vi "S8300E_CheckSN_auto.vi"() -> ()   [LabVIEW 2011]
panel:
  out "UUT SN":string
  out "UUT SN List":string
  out "CMD-LIST":cluster{string, string, string, string}[](array[cluster])
  out "log msg":string
  out "VISA resource name out":refnum<visa-resource-name>
  out "BEGIN TIME":u32
  out "進行狀況":string
  # "Error Code:SN-BIOS\nError Code:SN-DMI"
  # "S8300E Program SN (接UART COM9)"
  # "2014-12-12"
  # "Step1:Get Serial Number from BIOS Flash\nStep2:Get Serial Number from DMI table"
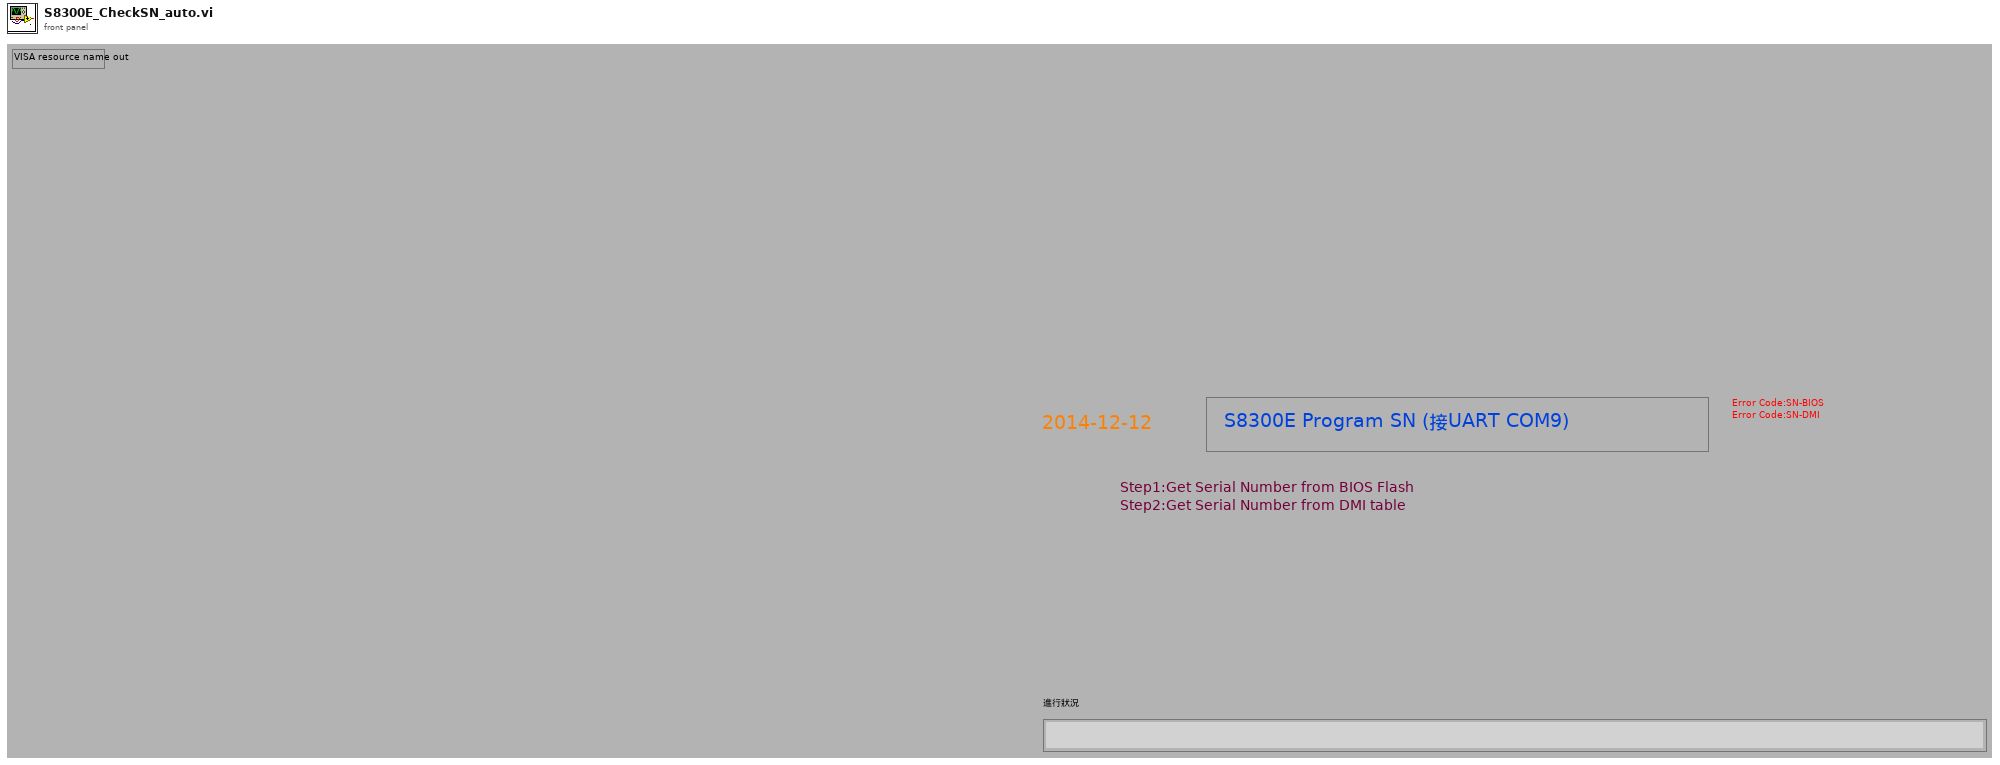
[diagram p1: front panel]
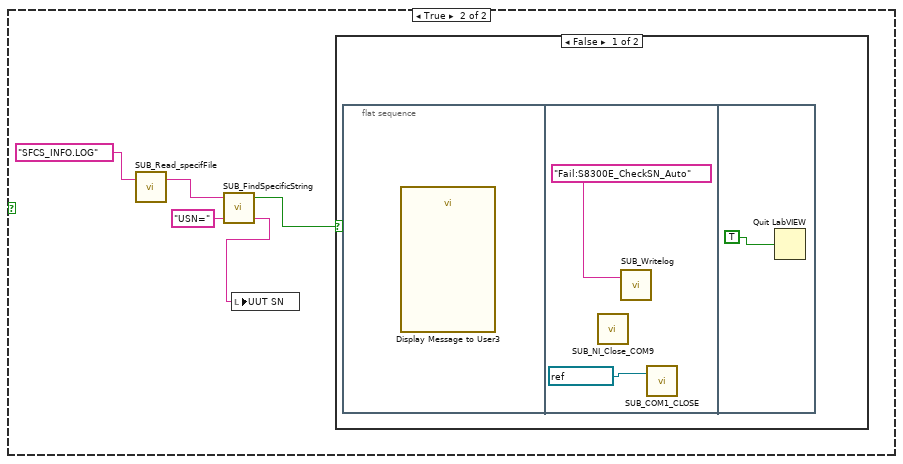
[diagram p3: hidden frame]
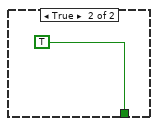
[diagram p8: hidden frame]
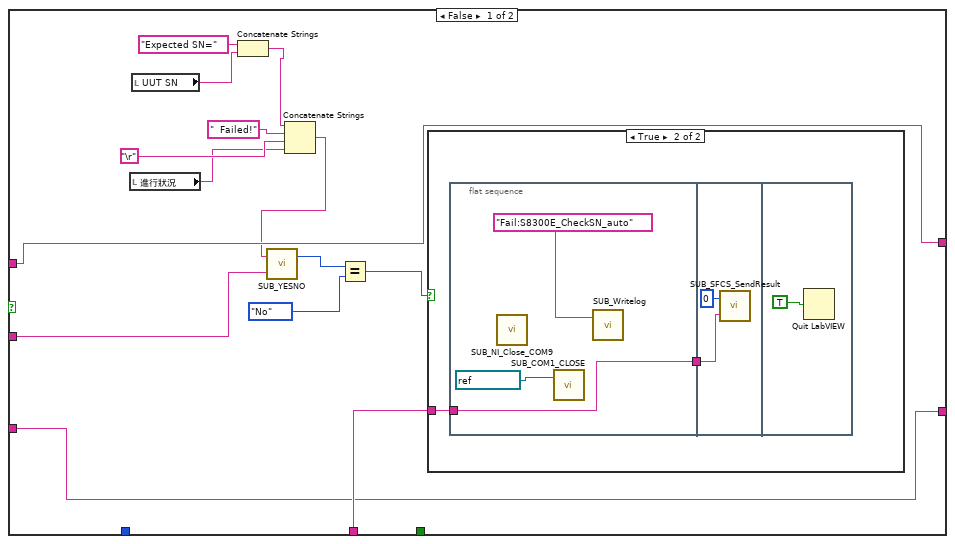
[diagram p9: hidden frame]
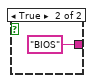
[diagram p11: hidden frame]
diagram:
  n1 = flat-sequence {
    frame #0 {
      n2 = Tick Count (ms)() -> (millisecond timer value=→"BEGIN TIME":u32)
    }
    frame #1 {
      n3 = call "SUB_COM1_CLOSE.vi"("VISA resource name"=refnum<visa-resource-name> "COM9") -> ()  [unwired: 3 in]
      n4 = call "SUB_COM1_CLOSE.vi"("VISA resource name"=refnum<visa-resource-name> "COM9") -> ()  [unwired: 3 in]
      n5 = property on="進行狀況" class="Str"("Blinking"=TRUE) -> ()  [unwired: 2 in, 2 out]
      "進行狀況" <- "進入測試準備中...." ("進行狀況")
      "UUT SN" <- ""
    }
    frame #2 {
      n6 = call "SUB_SearchFile_inFolder.vi"("Search Filename in Folder"="S8300E_sfcs_misc.txt") -> ("File Existing True/Flase"=w7:bool)  [unwired: 1 in]
      n7 = case shown="False" w7 {
        frame False {
          n8 = flat-sequence {
            frame #0 {
              n9 = call "Display Message to User"() -> ()  [unwired: 10 in, 2 out]
            }
            frame #1 {
              n10 = call "SUB_COM1_CLOSE.vi"("VISA resource name"=refnum<visa-resource-name> "COM9") -> ()  [unwired: 3 in]
              n11 = call "SUB_Writelog.vi"("Pass/Fail"="Fail:S8300E_CheckSN_Manual") -> ()  [unwired: 2 in]
            }
            frame #2 {
              n12 = Quit LabVIEW(quit? (T)=TRUE) -> ()
            }
          }
        }
        frame True {
        }
      }
    }
    frame #3 {
      n13 = call "SUB_SearchFile_inFolder.vi"("Search Filename in Folder"="SFCS_INFO.LOG") -> ("File Existing True/Flase"=w12:bool)  [unwired: 1 in]
      n14 = case shown="False" w12 {
        frame False {
          n15 = flat-sequence {
            frame #0 {
              n16 = call "Display Message to User2"() -> ()  [unwired: 10 in, 2 out]
            }
            frame #1 {
              n17 = call "SUB_Writelog.vi"("Pass/Fail"="Fail:S8300E_CheckSN_Auto") -> ()  [unwired: 2 in]
              n18 = call "SUB_NI_Close_COM9.vi"() -> ()  [unwired: 1 in, 1 out]
              n19 = call "SUB_COM1_CLOSE.vi"("VISA resource name"=refnum<visa-resource-name> "COM9") -> ()  [unwired: 3 in]
            }
            frame #2 {
              n20 = Quit LabVIEW(quit? (T)=TRUE ("stop? (T)")) -> ()
            }
          }
        }
        frame True {
          n21 = call "SUB_Read_specifFile.vi"("name or relative path"="SFCS_INFO.LOG") -> ("text"=w20:string)  [unwired: 1 in, 1 out]
          n22 = call "SUB_FindSpecificString.vi"("Find this String"="USN=", "String data"=w20) -> ("before \"; \" string"=w17:string, "Found"=w18:bool)  [unwired: 2 in]
          n23 = local write "UUT SN"(w17) -> ()
          n24 = case shown="False" w18 {
            frame False {
              n25 = flat-sequence {
                frame #0 {
                  n26 = call "Display Message to User3"() -> ()  [unwired: 10 in, 2 out]
                }
                frame #1 {
                  n27 = call "SUB_NI_Close_COM9.vi"() -> ()  [unwired: 1 in, 1 out]
                  n28 = call "SUB_Writelog.vi"("Pass/Fail"="Fail:S8300E_CheckSN_Auto") -> ()  [unwired: 2 in]
                  n29 = call "SUB_COM1_CLOSE.vi"("VISA resource name"=refnum<visa-resource-name> "COM9") -> ()  [unwired: 3 in]
                }
                frame #2 {
                  n30 = Quit LabVIEW(quit? (T)=TRUE ("stop? (T)")) -> ()
                }
              }
            }
            frame True {
            }
          }
        }
      }
    }
    frame #4 {
      n31 = local read "UUT SN"() -> (w26:string)
      n32 = Concatenate Strings("PASSED=", w26) -> (w25:string)
      n33 = Concatenate Strings("PASSED=", w26) -> (w28:string)
      n34 = Concatenate Strings("./ser.sh -w -f  ", w26, "\r") -> (w47:string)
      n35 = Concatenate Strings("./ser.sh -r -f  ", "\r") -> (w43:string)
      n36 = Concatenate Strings("./ser.sh -r -d ", "\r") -> (w40:string)
      n37 = Bundle(w47, "PASSED=", "Set Serial Number to BIOS Flash", "SN-BIOS") -> ()  [unwired: 1 in, 1 out]
      n38 = Bundle(w43, w28, "Get Serial Number from BIOS Flash", "SN-BIOS") -> (w35:cluster{string, string, string, string})  [unwired: 1 in]
      n39 = Bundle(w40, w25, "Get Serial Number from DMI table", "SN-DMI") -> (w34:cluster{string, string, string, string})  [unwired: 1 in]
      n40 = Build Array(w35, w34) -> (→"CMD-LIST":cluster{string, string, string, string}[])
    }
    frame #5 {
      n41 = case shown="True" TRUE {
        frame False {
        }
        frame True {
          n42 = call "SUB_COM9_INIT.vi"("baud rate"=u32 115200) -> ("VISA resource name out"=w53:refnum<visa-resource-name>)  [unwired: 1 in, 1 out]
          "VISA resource name out" <- w53
          n43 = call "SUB_COM1Wrt.vi"("VISA resource name"=w53, "write buffer"="\r") -> ("duplicate VISA resource name"=w50:refnum<visa-resource-name>)  [unwired: 1 in, 1 out]
          n44 = call "SUB_ContinueCom1Read.vi"("Numeric"=1200, "duplicate VISA resource name 2"=w50) -> ()  [unwired: 1 in, 3 out]
        }
      }
    }
    frame #6 {
      n45 = case shown="True" TRUE {
        frame False {
        }
        frame True {
          n46 = while {
            stop <- w65 stop-if-true
            w56 = "\r"
            n47 = Concatenate Strings(w56, w56, w56) -> (w57:string)
            n48 = local read "VISA resource name out"() -> (w58:refnum<visa-resource-name>)
            n49 = call "SUB_COM1Wrt.vi"("VISA resource name"=w58, "write buffer"=w57) -> ("duplicate VISA resource name"=w64:refnum<visa-resource-name>)  [unwired: 1 in, 1 out]
            n50 = Tick Count (ms)() -> (millisecond timer value=w63:u32)
            n51 = call "SUB_READ_COM1_FindString_timeout.vi"("Find this String"="s8300e_func_test#", "Timeout Seccond"=3.0, "Begin time"=w63, "duplicate VISA resource name 2"=w64) -> ("Output String"=w59:string, "Found String"=w60:bool)  [unwired: 1 in, 1 out]
            n52 = case shown="False" w60 {
              tunnel: [w67 TRUE] -> w65
              tunnel: w59 -> [w66 _]
              frame False {
                n53 = call "SUB_YESNO.vi"("Debug View"=w66, "Status"="UART無正確反應!需有S8300E字串") -> ("yes/no"=w70:enum32{"No Selection", "Yes", "No", "None"})  [unwired: 1 in]
                n54 = Equal?(x=w70, y=enum32{"No Selection", "Yes", "No", "None"}."No") -> (x = y?=w68:bool)
                n55 = case shown="True" w68 {
                  tunnel: [_ w72] -> w67
                  frame False {
                  }
                  frame True {
                    n56 = flat-sequence {
                      tunnel: [w77] -> w72
                      frame #0 {
                        n57 = call "SUB_Writelog.vi"("Pass/Fail"="Fail:S8300E_CheckSN_Manual") -> ()  [unwired: 2 in]
                        n58 = call "SUB_NI_Close_COM9.vi"() -> ()  [unwired: 1 in, 1 out]
                        n59 = call "SUB_COM1_CLOSE.vi"("VISA resource name"=refnum<visa-resource-name> "COM9") -> ()  [unwired: 3 in]
                      }
                      frame #1 {
                        n60 = call "SUB_SFCS_SendResult.vi"("ErrorCode"="UART", "PASS_Fail (1/0)"=i8 0) -> ()  [unwired: 1 out]
                      }
                      frame #2 {
                        w77 = TRUE ("quit? (T)")
                        n61 = Quit LabVIEW(quit? (T)=w77) -> ()
                      }
                    }
                  }
                }
              }
              frame True {
              }
            }
          }
        }
      }
    }
    frame #7 {
      n62 = local read "CMD-LIST"() -> (w81:cluster{string, string, string, string}[])
      n63 = Array Size(array=w81) -> (size(s)=w84:i32)
      n64 = for {
        N: w84 -> [_]
        shift-right: [w89] -> w82
        shift-left: "" -> [w88]
        shift-right: [w86] -> w79
        shift-left: "" -> [w85]
        i -> [w87]
        n65 = while {
          tunnel: w87 -> [w108]
          tunnel: [w100] -> w89
          tunnel: w88 -> [w99]
          tunnel: w87 -> [w92]
          tunnel: [w91] -> w86
          tunnel: w85 -> [w90]
          stop <- w102 stop-if-true
          n66 = local read "VISA resource name out"() -> (w104:refnum<visa-resource-name>)
          n67 = local read "CMD-LIST"() -> (w98:cluster{string, string, string, string}[])
          n68 = Index Array(array=w98, index=w108) -> (element=w97:cluster{string, string, string, string})
          n69 = Unbundle(w97) -> (w96:string, w94:string, w95:string, w93:string)
          n70 = call "SUB_COM1Wrt.vi"("VISA resource name"=w104, "write buffer"=w96) -> ("duplicate VISA resource name"=w107:refnum<visa-resource-name>)  [unwired: 1 in, 1 out]
          n71 = Tick Count (ms)() -> (millisecond timer value=w106:u32)
          n72 = call "SUB_READ_COM1_FindString_timeout.vi"("Find this String"=w94, "Timeout Seccond"=2.0, "Begin time"=w106, "duplicate VISA resource name 2"=w107) -> ("Output String"=w101:string, "Found String"=w103:bool)  [unwired: 1 in, 1 out]
          n73 = local write "進行狀況"(w95) -> ()
          n74 = case shown="True" w103 {
            tunnel: [_ TRUE] -> w102
            tunnel: w101 -> [w122 w140]
            tunnel: [w118 w144] -> w100
            tunnel: w99 -> [w118 w143]
            tunnel: w93 -> [w117 _]
            tunnel: w92 -> [_ w133]
            tunnel: [w112 w135] -> w91
            tunnel: w90 -> [w112 w134]
            frame False {
              n75 = local read "進行狀況"() -> (w114:string)
              n76 = local read "UUT SN"() -> (w110:string)
              n77 = Concatenate Strings("Expected SN=" ("string"), w110) -> (w109:string)
              n78 = Concatenate Strings(w109, "  Failed!" ("string"), "\r", w114) -> (w113:string)
              n79 = call "SUB_YESNO.vi"("Debug View"=w122, "Status"=w113) -> ("yes/no"=w121:enum32{"No Selection", "Yes", "No", "None"})  [unwired: 1 in]
              n80 = Equal?(x=w121, y=enum32{"No Selection", "Yes", "No", "None"}."No") -> (x = y?=w119:bool)
              n81 = case shown="True" w119 {
                tunnel: w117 -> [_ w123]
                frame False {
                }
                frame True {
                  n82 = flat-sequence {
                    tunnel: [w126] -> w124
                    tunnel: w123 -> [w126]
                    tunnel: w124 -> [w128]
                    frame #0 {
                      n83 = call "SUB_NI_Close_COM9.vi"() -> ()  [unwired: 1 in, 1 out]
                      n84 = call "SUB_COM1_CLOSE.vi"("VISA resource name"=refnum<visa-resource-name> "COM9") -> ()  [unwired: 3 in]
                      n85 = call "SUB_Writelog.vi"("Pass/Fail"="Fail:S8300E_CheckSN_auto") -> ()  [unwired: 2 in]
                    }
                    frame #1 {
                      n86 = call "SUB_SFCS_SendResult.vi"("ErrorCode"=w128, "PASS_Fail (1/0)"=i8 0) -> ()  [unwired: 1 out]
                    }
                    frame #2 {
                      n87 = Quit LabVIEW(quit? (T)=TRUE) -> ()
                    }
                  }
                }
              }
            }
            frame True {
              n88 = call "SUB_FindSpecificString.vi"("Find this String"="PASSED=", "String data"=w140) -> ("before \"; \" string"=w138:string)  [unwired: 2 in, 1 out]
              n89 = Equal To 0?(x=w133) -> (x = 0?=w132:bool)
              n90 = case shown="False" w132 {
                tunnel: ["DMI" ("string") "BIOS" ("string")] -> w131
                frame False {
                }
                frame True {
                }
              }
              n91 = Concatenate Strings("SN-" ("string"), w131, "=" ("string"), w138, "\r") -> (w136:string)
              n92 = Concatenate Strings(w143, w140) -> (w144:string)
              n93 = Concatenate Strings(w134, w136) -> (w135:string)
            }
          }
        }
      }
      "log msg" <- w82
      "UUT SN List" <- w79
    }
    frame #8 {
      w151 = "\n"
      n94 = local read "log msg"() -> (w152:string)
      n95 = local read "UUT SN List"() -> (w150:string)
      n96 = local read "BEGIN TIME"() -> (w156:u32)
      n97 = Tick Count (ms)() -> (millisecond timer value=w155:u32)
      n98 = call "SUB_CAL_TESTTIME.vi"("Test Item name"="S8300E_CheckSN_auto", "Stop tick time"=w155, "Start tick time"=w156) -> ("Test Time output"=w149:string)  [unwired: 2 in]
      n99 = call "SUB_COM1_CLOSE.vi"("VISA resource name"=refnum<visa-resource-name> "COM9") -> ()  [unwired: 3 in]
      n100 = Concatenate Strings("Pass:S8300E_CheckSN_auto", w151, w152, w151, w150, w149) -> (w154:string)
      n101 = call "SUB_Writelog.vi"("Pass/Fail"=w154) -> ()  [unwired: 2 in]
    }
    frame #9 {
      n102 = Request Deallocation(TRUE ("flag")) -> ()
    }
    frame #10 {
      n103 = Quit LabVIEW(quit? (T)=TRUE ("stop? (T)")) -> ()
    }
  }
